vi "Update Result.vi"(4 "sp time stamp":timestamp, 5 "Peaks":dbl[](array[numeric]) format="%#_4p", 6 "Good fit?":dbl[](array[numeric]) format="%#_4p", 7 "Best fit results":dbl[][](array[numeric]) format="%#_4p", 8 "error in (no error)":errorcluster, 9 "Peaks absolute time":dbl[](array[numeric]), 10 "File":refnum<class "Acquired Result.lvclass">, 11 "Resonance Detector in":refnum<class "Resonance Detector.lvclass">) -> (0 "error out":errorcluster, 2 "File out":refnum<class "Acquired Result.lvclass">, 3 "Resonance Detector out":refnum<class "Resonance Detector.lvclass">)   [LabVIEW 2018, in "Resonance Detector.lvclass"]
uses:
  Resonance Detector.lvclass
  C:/github/LabActor/Process Object/Process Object.lvclass
  NHMFL_Core/Libraries/Instruments/Results/Acquired Result/Acquired Result.lvclass
  NHMFL_Core/Libraries/Instruments/Results/Acquired Result/Acquired Result.lvclass/Acquired Result.ctl
  Process Object/Process Object.lvclass/Process Object.ctl
  NHMFL_Core/Libraries/Instruments/Results/Acquired Result/Write Channels.vi
  NHMFL_Core/Libraries/Instruments/Results/Acquired Result/Write Group.vi
  NHMFL_Core/Libraries/Instruments/Results/Acquired Result/Write Time group.vi
  NHMFL_Core/Libraries/Instruments/Results/Acquired Result/Write Time value.vi
  Process Object/Write Result.vi
  Process Object/Write Result ready.vi
  Read Line detector configuration.vi
panel:
  # "F0         dF     Ampl   Phase   Xbgrd   Ybgrd"
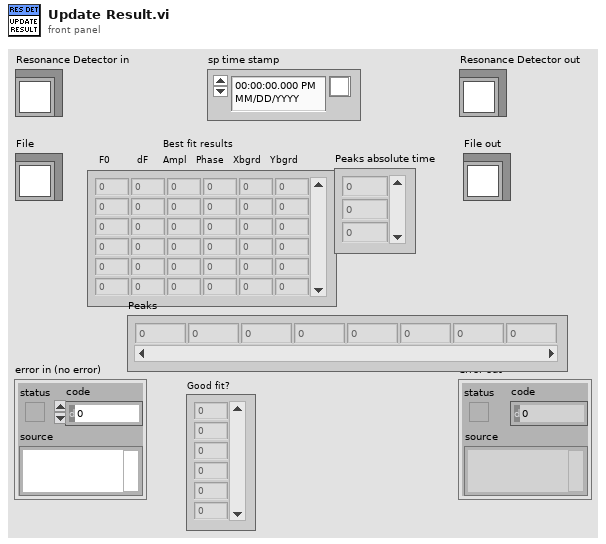
[diagram p1: front panel]
types:
  T1 = enum16{"open", "open or create", "create or replace", "create", "open (read-only)"}
  T2 = typedef "Line Detector Configuration.ctl" = cluster{"Peak width guess":dbl, "Background removal":enum16{"NONE", "High-pass", "Detrend"}, "Smoothing":enum16{"NONE", "Low-pass", "Denoise"}, "Smooth window":dbl, "Relative threshold":dbl, "Finder algorithm":enum16{"Basic", "Wavelet", "Wavelet+detrend"}, "Bgd window":dbl, "Spectrum recorder module name":string, "Fit window":dbl, "Initial fit guess":enum16{"Peak finder", "Last fit"}, "Follow\npeaks":bool, "Re-sample":dbl}
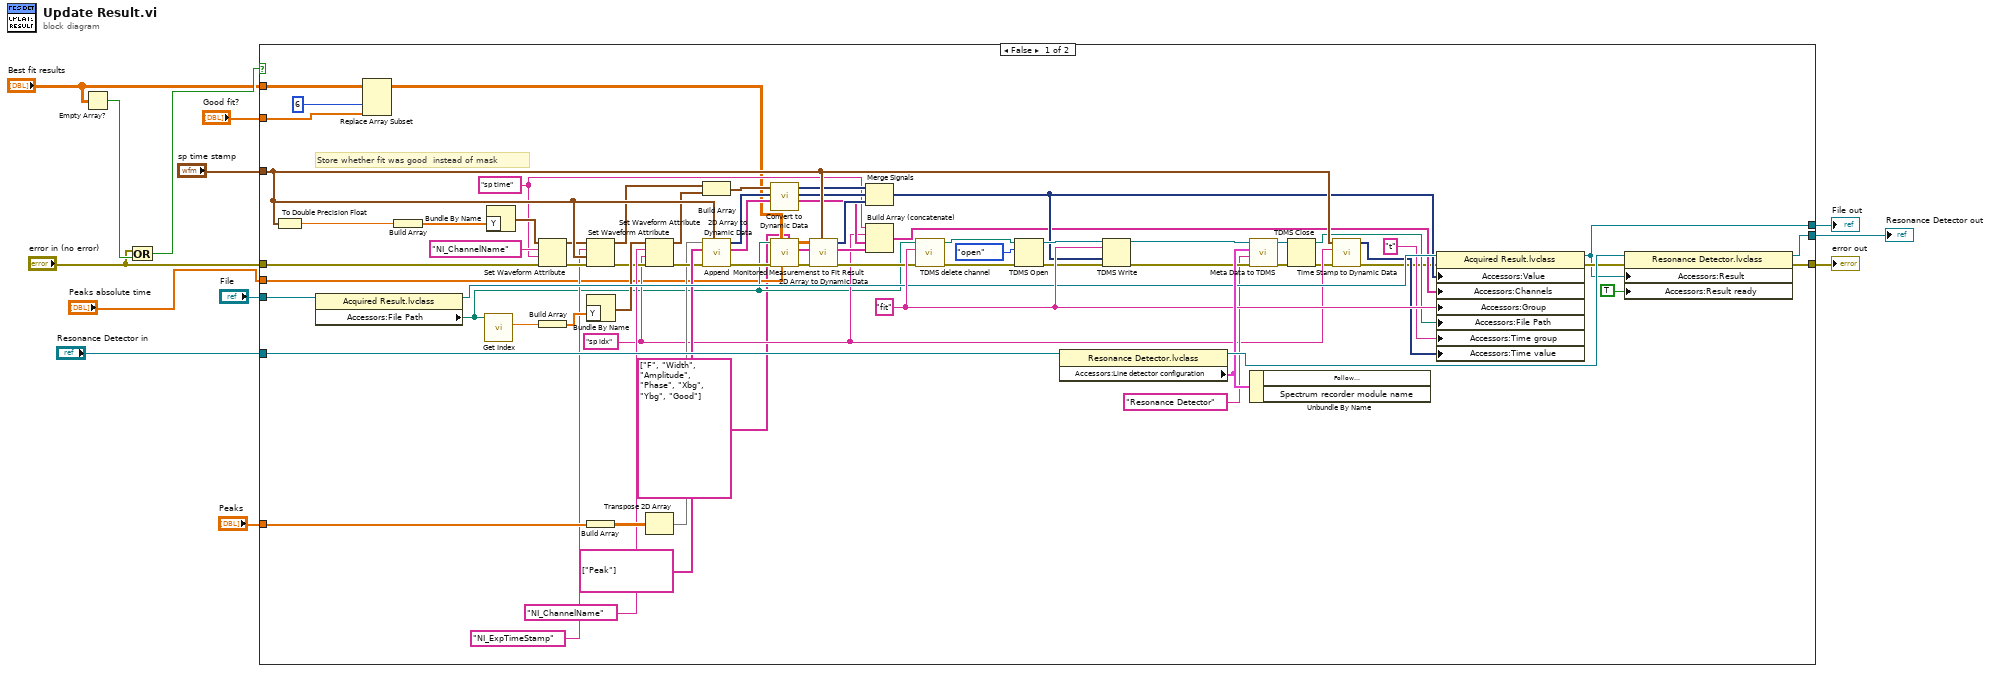
[diagram p0: block diagram]
diagram:
  n1 = Empty Array?(array="Best fit results") -> (empty?=w5:bool)
  n2 = Or(x="error in (no error)", y=w5) -> (x .or. y?=w7:bool)
  n3 = case shown="False" w7 {
    tunnel: [w22 w83] -> w13
    tunnel: [w23 w85] -> w11
    tunnel: "Resonance Detector in" -> [w77 w85]
    tunnel: "File" -> [w76 w84]
    tunnel: "Best fit results" -> [w25 _]
    tunnel: "Peaks" -> [w80 _]
    tunnel: "sp time stamp" -> [w79 _]
    tunnel: "error in (no error)" -> [w28 w83]
    tunnel: [w27 w84] -> w3
    tunnel: "Good fit?" -> [w24 _]
    tunnel: "Peaks absolute time" -> [w17 _]
    frame False {
      w51 = "sp time" ("name")
      w31 = "sp idx" ("name")
      w78 = "fit"
      # "Store whether fit was good  instead of mask"
      n4 = To Double Precision Float(number=w79) -> (double precision float=w52:dbl)
      n5 = property class="Acquired Result.lvclass"(reference=w76) -> (reference out=w75:refnum<class "Acquired Result.lvclass">, "Accessors:File Path"=w19:path)  [unwired: 1 in, 1 out]
      n6 = Replace Array Subset(array=w25, new element=w24, index (col)=6 ("disabled index (col)")) -> (w16:dbl[][])  [unwired: 1 in]
      n7 = Build Array(w52) -> (w33:dbl[])
      n8 = call "Get Index.vi"("File Path Control"=w19) -> ("DBL number"=w42:dbl)  [unwired: 9 in, 1 out]
      n9 = Bundle By Name("Y"=w33) -> (w54:waveform(dbl))  [unwired: 1 in]
      n10 = Set Waveform Attribute(4:w28, 5:w51, 6:"NI_ChannelName" ("name"), 7:w54) -> (0:w40:errorcluster, 3:w39:waveform(dbl))  [unwired: 1 out]
      n11 = Build Array(w42) -> (w63:dbl[])
      n12 = Set Waveform Attribute(4:w40, 5:w79, 6:"NI_ExpTimeStamp" ("name"), 7:w39) -> (0:w37:errorcluster, 3:w38:waveform(dbl))  [unwired: 1 out]
      n13 = Bundle By Name("Y"=w63) -> (w62:waveform(dbl))  [unwired: 1 in]
      n14 = Build Array(w80) -> (w69:dbl[][])
      n15 = Set Waveform Attribute(4:w37, 5:w31, 6:"NI_ChannelName" ("name"), 7:w62) -> (0:w60:errorcluster, 3:w34:waveform(dbl))  [unwired: 1 out]
      n16 = Transpose 2D Array(2D array=w69) -> (transposed array=w55:dbl[][])
      n17 = Build Array(w38, w34) -> (w59:waveform(dbl)[])
      n18 = call "2D Array to Dynamic Data.vi"("Time Stamp Control"=w79, "Error In"=w60, "Channels"=string[] ["Peak"], "Array"=w55) -> ("Error Out"=w21:errorcluster, "Channels out"=w65:string[], "Dynamic Data Type"=w68:dynamicdata)  [unwired: 5 in]
      n19 = call "Convert to Dynamic Data"("Array of Waveforms"=w59) -> ("Dynamic Data Type"=w58:dynamicdata)  [unwired: 3 in]
      n20 = call "Append  Monitored Measuremenst to Fit Result.vi"("Channels"=string[] ["F", "Width", "Amplitude", "Phase", "Xbg", "Ybg", "Good"], "Peaks absolute time"=w17, "Data in"=w16, "Error In"=w21, "file path"=w19) -> ("Error Out"=w20:errorcluster, "Channels out"=w18:string[], "Data out"=w15:dbl[][])  [unwired: 4 in]
      n21 = call "2D Array to Dynamic Data.vi"("Time Stamp Control"=w79, "Error In"=w20, "Channels"=w18, "Array"=w15) -> ("Error Out"=w45:errorcluster, "Channels out"=w64:string[], "Dynamic Data Type"=w67:dynamicdata)  [unwired: 5 in]
      n22 = Merge Signals(w58, w68, w67) -> (w57:dynamicdata)
      n23 = Build Array (concatenate)(w51, w31, w65, w64) -> (w56:string[])
      n24 = call "TDMS delete channel.vi"("error in (no error)"=w45, "group name"=w78, "file path"=w19) -> ("error out"=w73:errorcluster, "file path out"=w72:path)  [unwired: 6 in, 1 out]
      n25 = TDMS Open(8:w73, 10:T1."open" ("operation (0:open)"), 11:w72) -> (0:w71:errorcluster, 3:w70:refnum<k34>)  [unwired: 4 in]
      n26 = property class="Resonance Detector.lvclass"(reference=w77) -> (reference out=w82:refnum<class "Resonance Detector.lvclass">, "Accessors:Line detector configuration"=w81:T2)  [unwired: 1 in, 1 out]
      n27 = TDMS Write(0:w70, 5:w78, 9:w57, 11:w71) -> (4:w48:refnum<k34>, 15:w50:errorcluster)  [unwired: 2 in, 2 out]
      n28 = call "Meta Data to TDMS.vi"("Error In"=w50, "Name"="Resonance Detector", "Value"=w81, "tdms file"=w48) -> ("Error Out"=w49:errorcluster, "tdms file out"=w47:refnum<k34>)  [unwired: 6 in]
      n29 = Unbundle By Name(w81) -> ()  [unwired: 2 out]
      n30 = TDMS Close(8:w49, 11:w47) -> (0:w30:errorcluster, 3:w43:path)
      n31 = call "Time Stamp to Dynamic Data.vi"("Error In"=w30, "Name"=w31, "Time Stamp Control"=w79) -> ("Error Out"=w29:errorcluster, "Dynamic Data Type"=w32:dynamicdata)  [unwired: 7 in]
      n32 = property class="Acquired Result.lvclass"(reference=w75, error in=w29, "Accessors:Value"=w57, "Accessors:Channels"=w56, "Accessors:Group"=w78, "Accessors:File Path"=w43, "Accessors:Time group"="t" ("Time group"), "Accessors:Time value"=w32) -> (reference out=w27:refnum<class "Acquired Result.lvclass">, error out=w44:errorcluster)
      n33 = property class="Resonance Detector.lvclass"(reference=w82, error in=w44, "Accessors:Result"=w27, "Accessors:Result ready"=TRUE ("Result ready")) -> (reference out=w23:refnum<class "Resonance Detector.lvclass">, error out=w22:errorcluster)
    }
    frame True {
    }
  }
  "error out" <- w13
  "Resonance Detector out" <- w11
  "File out" <- w3
